vi "Light Color Read.vi"(8 "error in (no error)":errorcluster, 11 "3D Plot.lvclass in":refnum<class "3D Plot.lvclass">) -> (0 "error out":errorcluster, 1 "Light Color":u32, 3 "3D Plot.lvclass out":refnum<class "3D Plot.lvclass">)   [LabVIEW 2020, in "3D Plot.lvclass"]
uses:
  3D Plot.lvclass
  3D Plot.lvclass/3D Plot.ctl
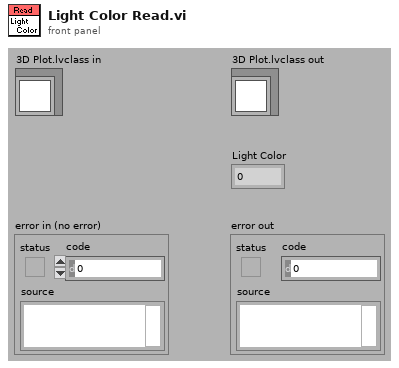
[diagram p1: front panel]
types:
  T1 = typedef "3D Plot.lvclass/Light Specific.ctl" = cluster{"Enable Light?":bool, "Light Color":u32, "Light Latitude":sgl, "Light Longitude":sgl, "Light Distance":sgl, "Attenuation":enum16{"None", "Linear", "Quadratic"}}
  T2 = enum16{"Light 0", "Light 1", "Light 2", "Light 3"}
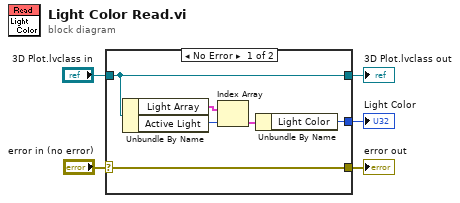
[diagram p0: block diagram]
diagram:
  n1 = case shown="No Error" "error in (no error)" {
    selector: "error in (no error)" -> [w6 w13]
    tunnel: [w11 _] -> w5
    tunnel: "3D Plot.lvclass in" -> [w7 w12]
    tunnel: [w7 w12] -> w3
    tunnel: [w6 w13] -> w1
    frame No Error {
      n2 = Unbundle By Name(w7) -> ("Light Array"=w8:T1[], "Active Light"=w9:T2)
      n3 = Index Array(array=w8, index=w9) -> (element=w10:T1)
      n4 = Unbundle By Name(w10) -> ("Light Color"=w11:u32)
    }
    frame Error {
    }
  }
  "error out" <- w1
  "Light Color" <- w5
  "3D Plot.lvclass out" <- w3
